vi "Write fit presets.vi"(0 "Config file in":T1, 5 "Fit parameters":T3={"A"=0.572086, "S"=0.0835606, "M1"=140.286, "M2"=140.486}, 7 "Physical constants":T2={"T1e (s)"=0.03, "T1n (s)"=1500.0}, 9 "C":dbl, 11 "error in (no error)":errorcluster) -> (4 "Config file out":T1, 15 "error out":errorcluster)   [LabVIEW 2019]
uses:
  Fit Parameters.ctl
  Physical Constants.ctl
  <vilib>/Utility/config.llb/Config Data RefNum.ctl
  <vilib>/Utility/config.llb/Write Key (Double).vi
  <vilib>/Utility/config.llb/NI_LVConfig.lvlib
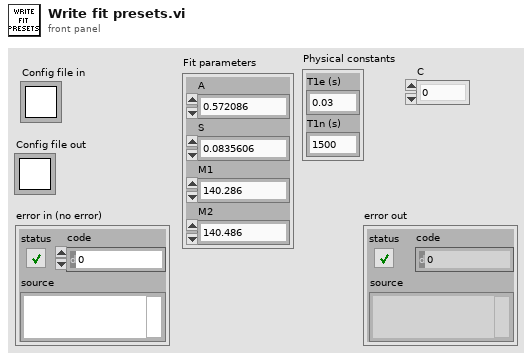
[diagram p1: front panel]
types:
  T1 = typedef "NI_LVConfig.lvlib/Config Data RefNum.ctl" = refnum<k1>
  T2 = typedef "Physical Constants.ctl" = cluster{"T1e (s)":dbl, "T1n (s)":dbl}
  T3 = typedef "Fit Parameters.ctl" = cluster{"A":dbl, "S":dbl, "M1":dbl, "M2":dbl}
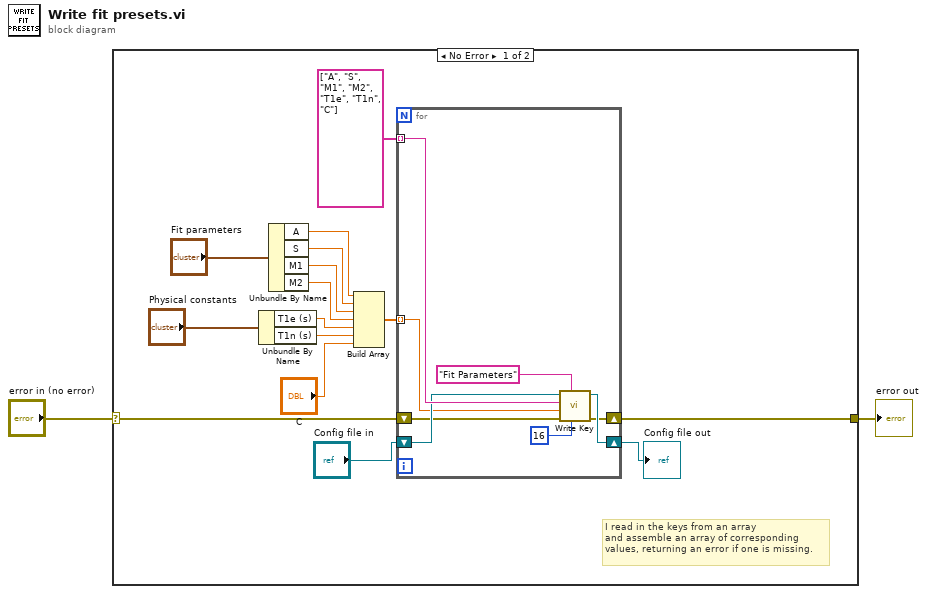
[diagram p0: block diagram]
diagram:
  n1 = case shown="No Error" "error in (no error)" {
    selector: "error in (no error)" -> [w4 w26]
    tunnel: [w3 w26] -> w1
    frame No Error {
      # "I read in the keys from an array\nand assemble an array of corresponding\nvalues, returning an error if one is missing."
      n2 = Unbundle By Name("Physical constants") -> ("T1e (s)"=w8:dbl, "T1n (s)"=w7:dbl)
      n3 = Unbundle By Name("Fit parameters") -> ("A"=w12:dbl, "S"=w11:dbl, "M1"=w10:dbl, "M2"=w9:dbl)
      n4 = Build Array(w12, w11, w10, w9, w8, w7, "C") -> (w5:dbl[])
      n5 = for {
        tunnel: string[] ["A", "S", "M1", "M2", "T1e", "T1n", "C"] -> [w25] mode=indexing
        shift-right: [w22] -> w15
        shift-left: "Config file in" -> [w23]
        tunnel: w5 -> [w21] mode=indexing
        shift-right: [w18] -> w3
        shift-left: w4 -> [w19]
        n6 = call-poly <vilib>:"Write Key.vi"("precision (6)"=i16 16, "section"="Fit Parameters", "error in (no error)"=w19, "value"=w21, "key"=w25, "refnum"=w23) -> ("error out"=w18:errorcluster, "refnum out"=w22:T1)  [unwired: 3 in, 1 out]
      }
      "Config file out" <- w15
    }
    frame Error {
    }
  }
  "error out" <- w1
